vi "Read Translator.vi"(8 "error in (no error)":errorcluster, 11 "Observer.lvclass in":refnum<class "Observer.lvclass">) -> (0 "error out":errorcluster, 2 "Messenging.lvlib:Translator.lvclass":refnum<class "Translator.lvclass">, 3 "Observer.lvclass out":refnum<class "Observer.lvclass">)   [LabVIEW 2011, in "Messenging.lvlib" / "Observer.lvclass"]
uses:
  Observer.lvclass
  Message Translation/Translator/Translator.lvclass
  Observer.lvclass/Observer.ctl
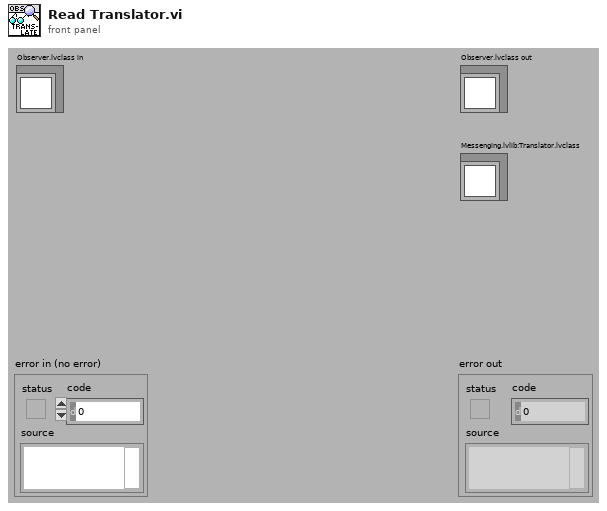
[diagram p1: front panel]
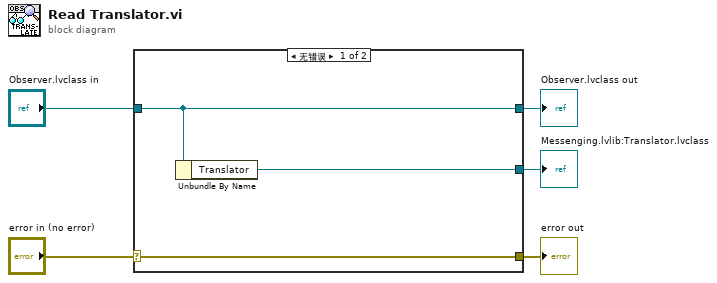
[diagram p0: block diagram]
diagram:
  n1 = case shown="无错误" "error in (no error)" {
    selector: "error in (no error)" -> [w8 w9]
    tunnel: [w8 w9] -> w4
    tunnel: [w7 w10] -> w2
    tunnel: "Observer.lvclass in" -> [w7 w10]
    tunnel: [w6 _] -> w1
    frame No Error {
      n2 = Unbundle By Name(w7) -> ("Translator"=w6:refnum<class "Translator.lvclass">)
    }
    frame Error {
    }
  }
  "error out" <- w4
  "Observer.lvclass out" <- w2
  "Messenging.lvlib:Translator.lvclass" <- w1
